vi "Cost.vi"(8 "error in (no error)":errorcluster, 11 "Espresso in":refnum<class "House Blend.lvclass">) -> (0 "error out":errorcluster, 2 "Cost":dbl, 3 "Espresso out":refnum<class "House Blend.lvclass">)   [LabVIEW 2011, in "House Blend.lvclass"]
uses:
  House Blend.lvclass
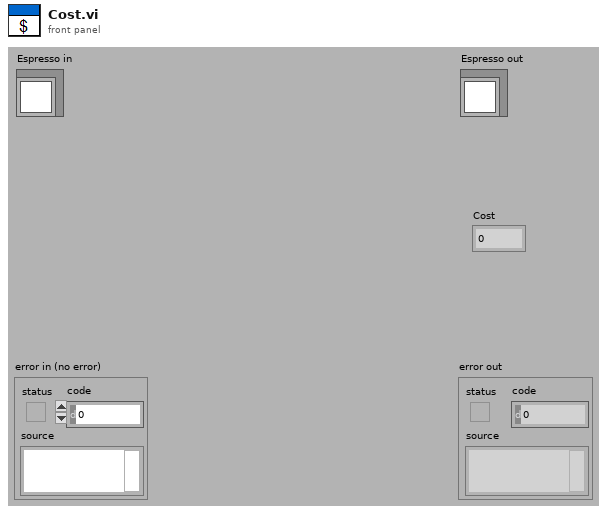
[diagram p1: front panel]
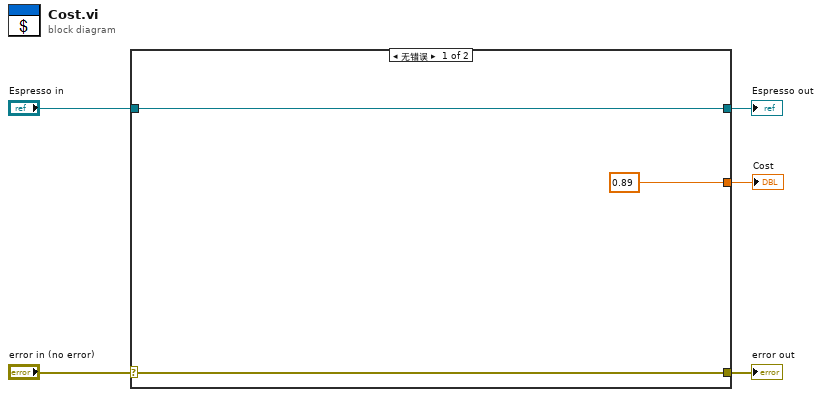
[diagram p0: block diagram]
diagram:
  n1 = case shown="无错误" "error in (no error)" {
    selector: "error in (no error)" -> [w7 w10]
    tunnel: [w7 w10] -> w4
    tunnel: [w8 w9] -> w2
    tunnel: "Espresso in" -> [w8 w9]
    tunnel: [0.89 ("Cost") _] -> w1
    frame No Error {
    }
    frame Error {
    }
  }
  "error out" <- w4
  "Espresso out" <- w2
  "Cost" <- w1
